vi "niRFUtil FTW Generate Mean Average FIR Filter.vi"(2 "Sampling Rate (Hz)":dbl=500000.0 format="%^.3e", 3 "Samples":i32=5) -> (1 "Filter":T1 {"y" min=0 max=127 format="%.2f"; "dx" format="%^.2e"; "x0" format="%^.2e"})   [LabVIEW 2015, in "niRFUtil.lvlib"]
doc: "(c) Copyright 2006, National Instruments, Inc. This VI may not be duplicated, sold, or distributed without written consent from National Instruments."
uses:
  niRFUtil.lvlib
  Includes/niRFUtil INC Real Waveform.ctl
  Includes/niRFUtil INC Real Array.ctl
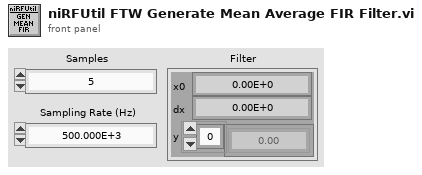
[diagram p1: front panel]
types:
  T1 = typedef "niRFUtil.lvlib/niRFUtil INC Real Waveform.ctl" = cluster{"x0":dbl, "dx":dbl, "y":T2}
  T2 = typedef "niRFUtil.lvlib/niRFUtil INC Real Array.ctl" = sgl[]
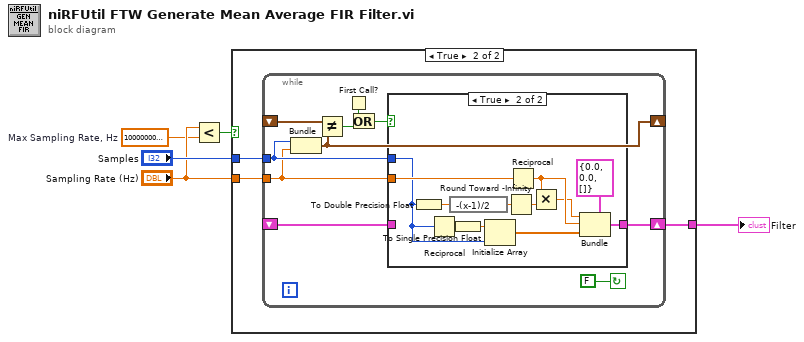
[diagram p0: block diagram]
diagram:
  w1 = 1000000000.0  # Max Sampling Rate, Hz
  n1 = Less?(x="Sampling Rate (Hz)", y=w1) -> (x < y?=w3:bool)
  n2 = case shown="True" w3 {
    tunnel: "Sampling Rate (Hz)" -> [_ w8]
    tunnel: [_ w7] -> w5
    tunnel: "Samples" -> [_ w6]
    frame False {
    }
    frame True {
      n3 = while {
        shift-right: [w17] -> w7
        shift-left: _ -> [w16]
        tunnel: w8 -> [w10]
        shift-right: [w9] -> _
        shift-left: _ -> [w15]
        tunnel: w6 -> [w11]
        stop <- FALSE continue-if-true
        n4 = Bundle("Samples"=w11, "Sampling Rate (Hz)"=w10) -> (w9:cluster{"Samples":i32, "Sampling Rate (Hz)":dbl})  [unwired: 1 out]
        n5 = Not Equal?(x=w15, y=w9) -> (x != y?=w12:bool)
        n6 = First Call?() -> (First Call?: T/F=w14:bool)
        n7 = Or(x=w14, y=w12) -> (x .or. y?=w13:bool)
        n8 = case shown="True" w13 {
          tunnel: [w19 w30] -> w17
          tunnel: w16 -> [w19 _]
          tunnel: w10 -> [_ w31]
          tunnel: w11 -> [_ w25]
          frame False {
          }
          frame True {
            n9 = To Double Precision Float(number=w25) -> (double precision float=w26:dbl)
            n10 = Reciprocal(x=w25) -> (1/x=w24:dbl)
            n11 = expression code="-(x-1)/2"(w26) -> (w29:dbl)
            n12 = To Single Precision Float(number=w24) -> (single precision float=w20:sgl)
            n13 = Initialize Array(w20, w25) -> (w22:sgl[])
            n14 = Round Toward -Infinity(1:w29) -> (0:w23:dbl)
            n15 = Reciprocal(x=w31) -> (1/x=w28:dbl)
            n16 = Multiply(x=w28, y=w23) -> (x*y=w27:dbl)
            n17 = Bundle(cluster=T1 {"x0"=0.0, "dx"=0.0, "y"=[]} ("Filter"), "x0"=w27, "dx"=w28, "y"=w22) -> (w30:T1)
          }
        }
      }
    }
  }
  "Filter" <- w5
